vi "SC TCP Open Sequence.vi"(8 "error in (no error)":errorcluster, 10 "Sequence":path, 11 "TCP Network Connection in":refnum<k5>) -> (0 "error out":errorcluster, 3 "TCP Network Connection out":refnum<k5>)   [LabVIEW 2018]
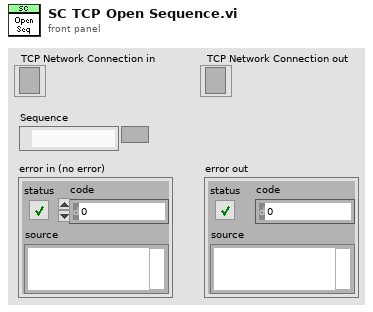
[diagram p1: front panel]
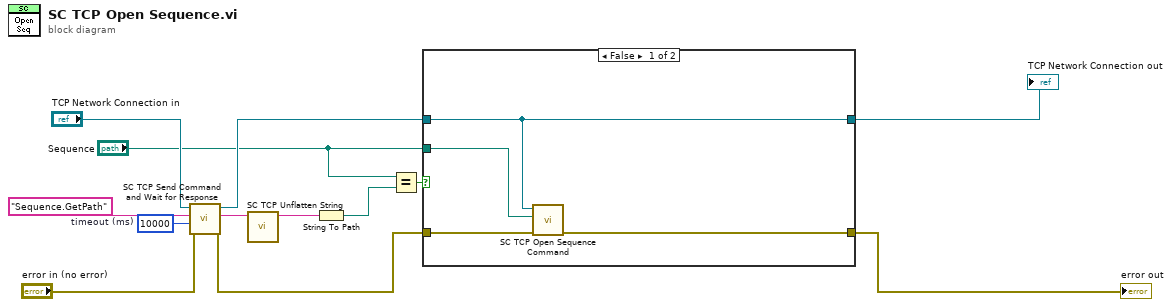
[diagram p0: block diagram]
diagram:
  w10 = 10000  # timeout (ms)
  n1 = call "SC TCP Send Command and Wait for Response.vi"("error in (no error)"="error in (no error)", "timeout (10000 ms)"=w10, "Command"="Sequence.GetPath", "TCP Network Connection in"="TCP Network Connection in") -> ("error out"=w4:errorcluster, "Response"=w8:string, "TCP Network Connection out"=w6:refnum<k5>)  [unwired: 4 in, 1 out]
  n2 = call "SC TCP Unflatten String.vi"("Response JSON"=w8) -> ("Return Data"=w3:string)  [unwired: 8 in, 2 out]
  n3 = String To Path(string=w3) -> (path=w1:path)
  n4 = Equal?(x="Sequence", y=w1) -> (x = y?=w12:bool)
  n5 = case shown="False" w12 {
    tunnel: w6 -> [w16 w18]
    tunnel: w4 -> [w15 w19]
    tunnel: [w14 w19] -> w11
    tunnel: "Sequence" -> [w17 _]
    tunnel: [w16 w18] -> w13
    frame False {
      n6 = call "SC TCP Open Sequence Command.vi"("error in (no error)"=w15, "Sequence to run (full path)"=w17, "TCP Network Connection in"=w16) -> ("error out"=w14:errorcluster)  [unwired: 7 in, 1 out]
    }
    frame True {
      # "Sequence didn't change since last time one was opened."
    }
  }
  "TCP Network Connection out" <- w13
  "error out" <- w11
